vi "array.vi"() -> ()   [LabVIEW 2017]
panel:
  out "Array":T1(array[cluster])
  out "1h avg 2":dbl[][](array[numeric])
  out "24h avg":dbl[][](array[numeric])
  out "Etykiety P1-6":string[][](array[string])
  out "wartosci":i32[](array[numeric])
  out "labels":i32[](array[numeric])
  in  "1h avg":dbl[][](array[numeric])
  out "FuelData":bool
  in  "AvgFuelLabels":T2
  in  "array 2":variant[](array[variant])
  in  "Avg fuel":T3
  in  "dummy fuel array":dbl[][][](array[numeric])
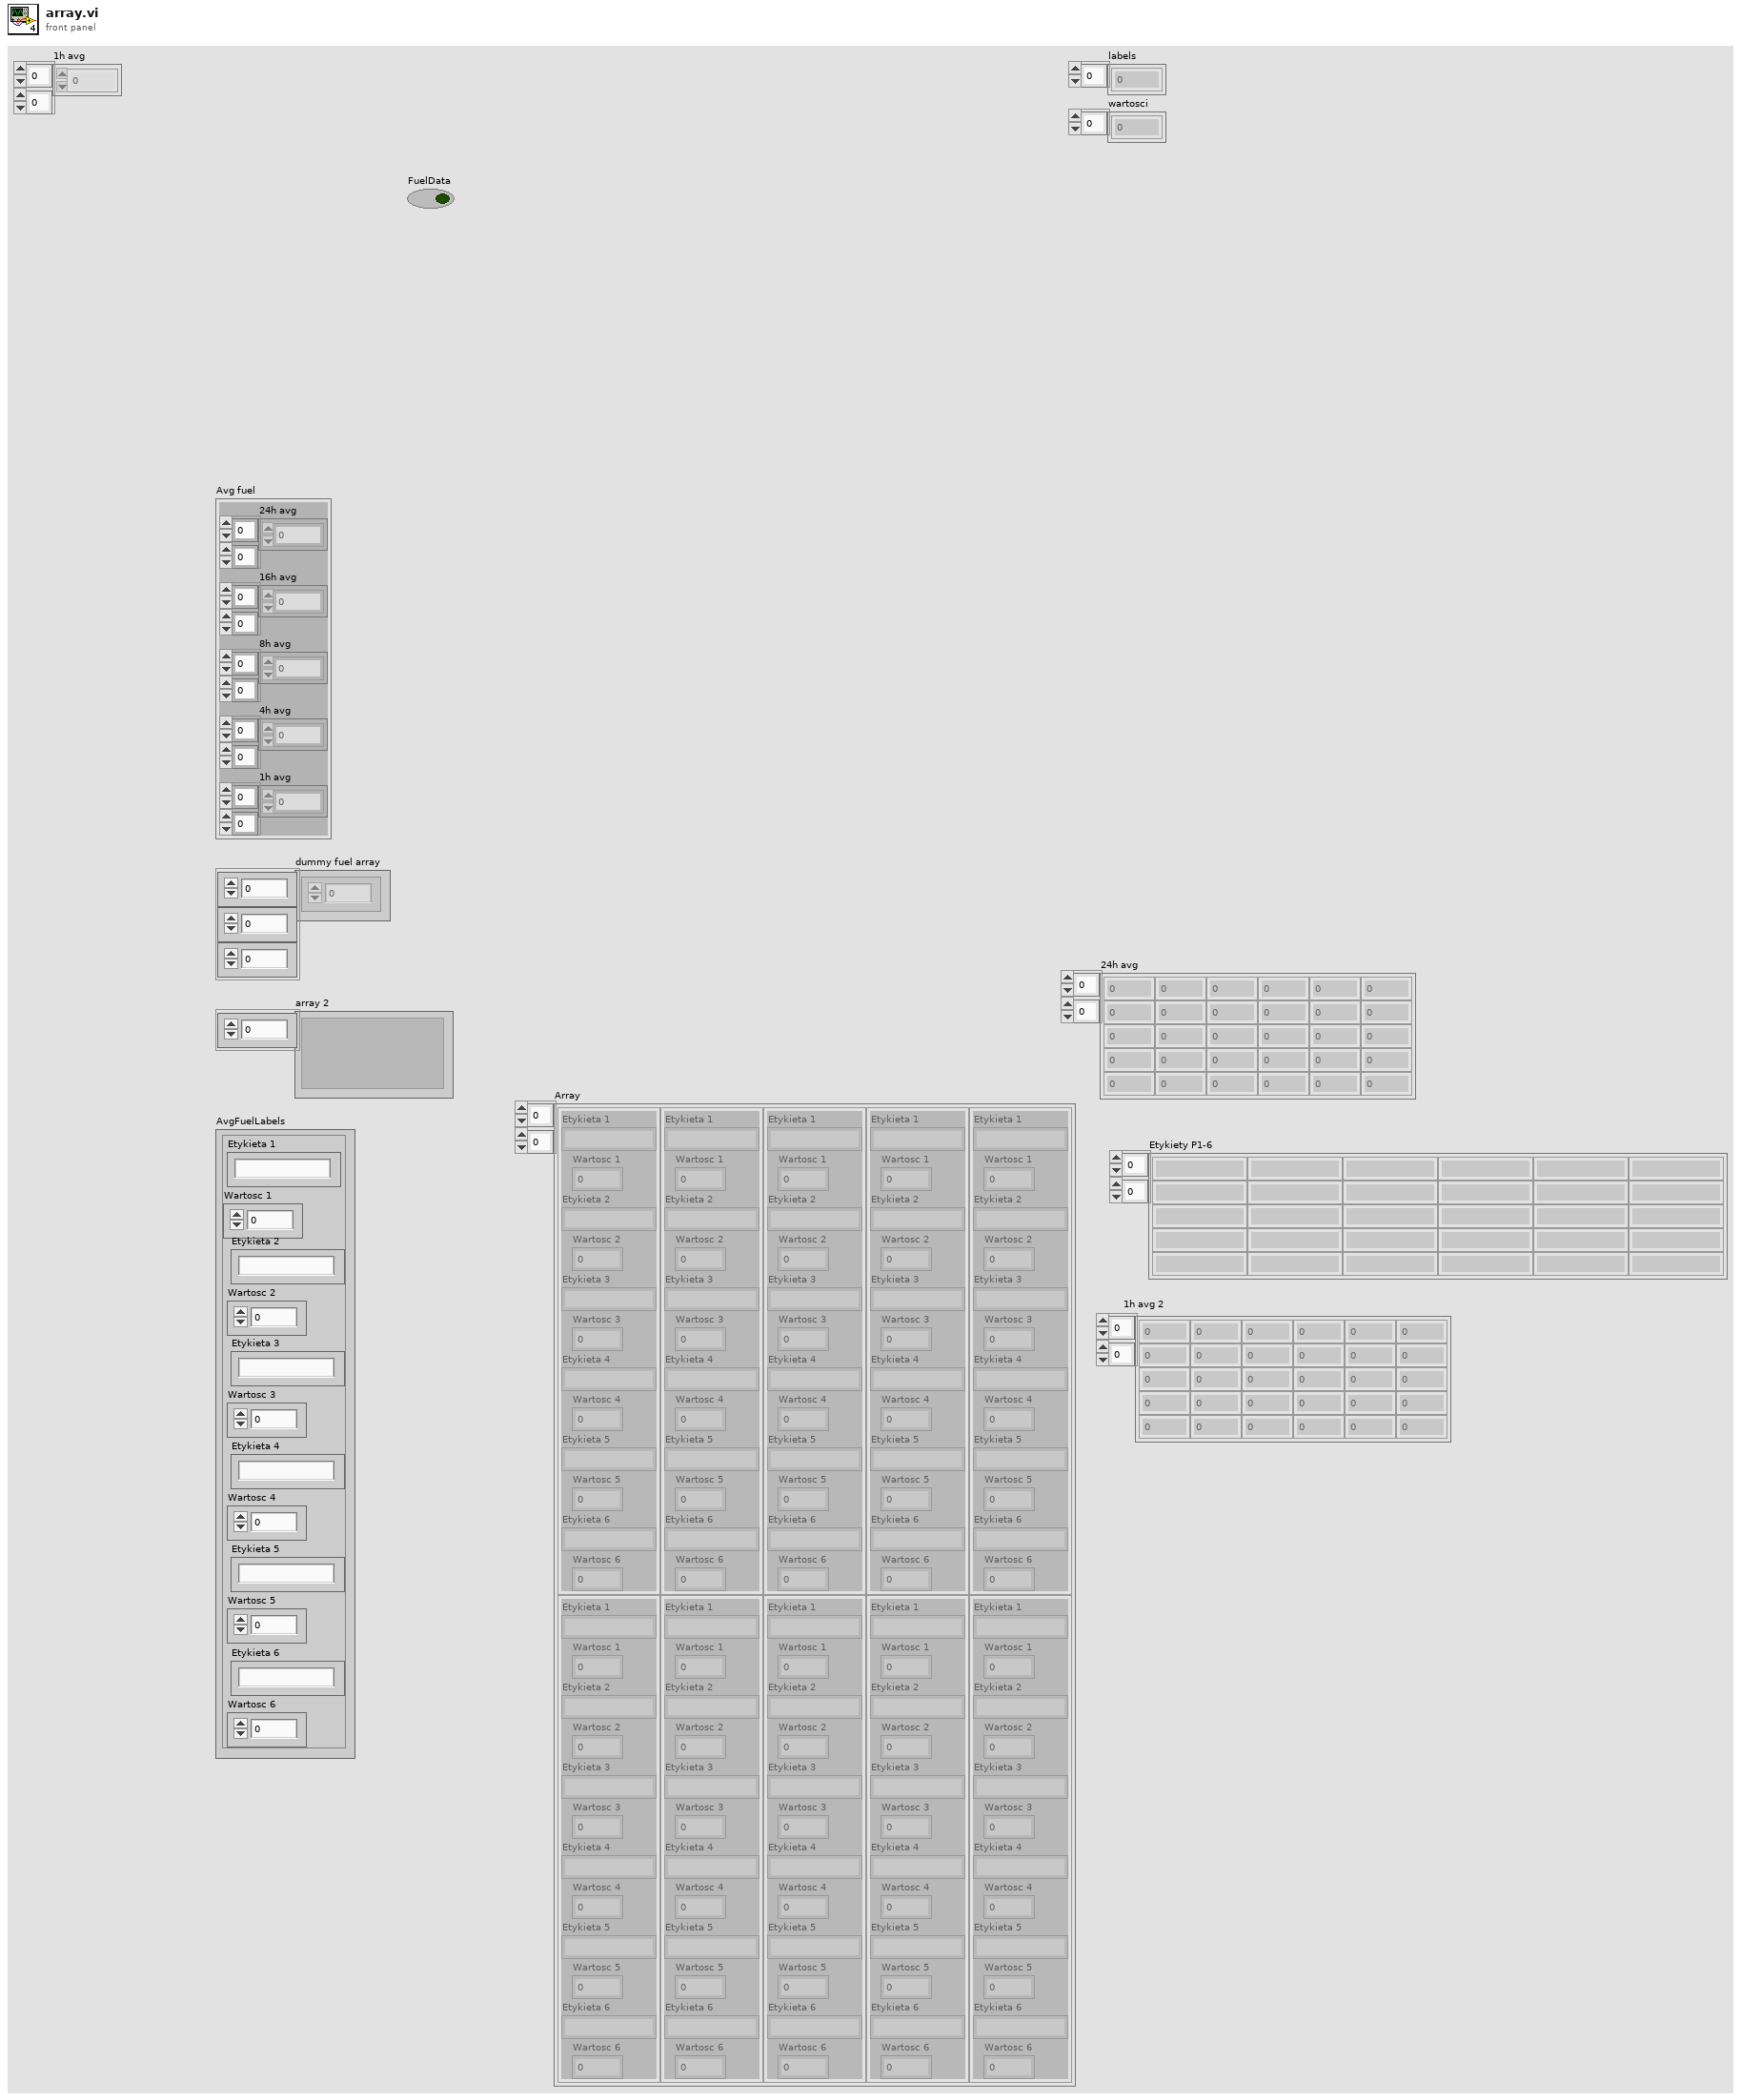
[diagram p1: front panel]
types:
  T1 = cluster{"Etykieta 1":string, "Wartosc 1":dbl, "Etykieta 2":string, "Wartosc 2":dbl, "Etykieta 3":string, "Wartosc 3":dbl, "Etykieta 4":string, "Wartosc 4":dbl, "Etykieta 5":string, "Wartosc 5":dbl, "Etykieta 6":string, "Wartosc 6":dbl}[][]
  T2 = cluster{"Etykieta 1":string, "Wartosc 1":dbl, "Etykieta 2":string, "Wartosc 2":dbl, "Etykieta 3":string, "Wartosc 3":dbl, "Etykieta 4":string, "Wartosc 4":dbl, "Etykieta 5":string, "Wartosc 5":dbl, "Etykieta 6":string, "Wartosc 6":dbl}
  T3 = cluster{"24h avg":dbl[][], "16h avg":dbl[][], "8h avg":dbl[][], "4h avg":dbl[][], "1h avg":dbl[][]}
  T4 = cluster{"Paliwo 1":string, "Paliwo 2":string, "Paliwo 3":string, "Paliwo 4":string, "Paliwo 5":string, "Paliwo 6":string}
  T5 = cluster{"array 2[0]":variant, "array 2[1]":variant, "array 2[2]":variant, "array 2[3]":variant, "array 2[4]":variant, "array 2[5]":variant, "array 2[6]":variant, "array 2[7]":variant, "array 2[8]":variant, "array 2[9]":variant, "array 2[10]":variant, "array 2[11]":variant}
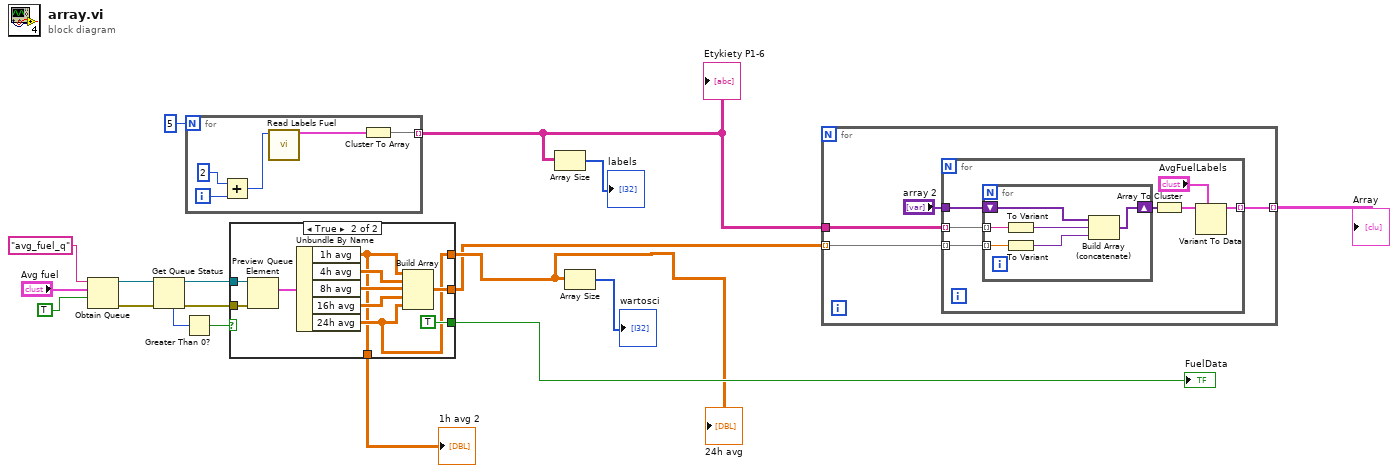
[diagram p0: block diagram]
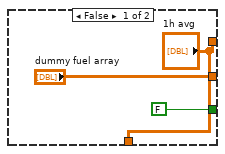
[diagram p2: hidden frame]
diagram:
  n1 = Obtain Queue(name (unnamed)="avg_fuel_q", element data type="Avg fuel", create if not found? (T)=TRUE) -> (queue out=w14:refnum<queue>, error out=w15:errorcluster)  [unwired: 2 in, 1 out]
  n2 = Get Queue Status(queue=w14, error in (no error)=w15) -> (queue out=w12:refnum<queue>, error out=w11:errorcluster, # elements in queue=w9:i32)  [unwired: 1 in, 5 out]
  n3 = Greater Than 0?(x=w9) -> (x > 0?=w10:bool)
  n4 = for {
    N: 5 -> [_]
    tunnel: [w20] -> w4 mode=indexing
    i -> [w23]
    n5 = Add(x=2, y=w23) -> (x+y=w21:i32)
    n6 = call "Read Labels Fuel.vi"("Slave ID"=w21) -> ("Etykiety P1-6"=w19:T4)  [unwired: 10 in]
    n7 = Cluster To Array(cluster=w19) -> (array=w20:string[])
  }
  "Etykiety P1-6" <- w4
  n8 = case shown="True" w10 {
    tunnel: w12 -> [_ w36]
    tunnel: w11 -> [_ w35]
    tunnel: [FALSE TRUE] -> w16
    tunnel: ["dummy fuel array" w33] -> w2
    tunnel: ["1h avg" w28] -> w3
    tunnel: ["1h avg" w27] -> w1
    frame False {
    }
    frame True {
      n9 = Preview Queue Element(queue=w36, error in (no error)=w35) -> (element=w32:T3)  [unwired: 1 in, 3 out]
      n10 = Unbundle By Name(w32) -> ("1h avg"=w27:dbl[][], "4h avg"=w30:dbl[][], "8h avg"=w31:dbl[][], "16h avg"=w29:dbl[][], "24h avg"=w28:dbl[][])
      n11 = Build Array(w27, w30, w31, w29, w28) -> (w33:dbl[][][])
    }
  }
  "FuelData" <- w16
  "24h avg" <- w3
  "1h avg 2" <- w1
  n12 = Array Size(array=w4) -> (size(s)=→"labels":i32[])
  n13 = Array Size(array=w3) -> (size(s)=→"wartosci":i32[])
  n14 = for {
    tunnel: [w40] -> w7 mode=indexing
    tunnel: w4 -> [w38]
    tunnel: w2 -> [w37] mode=indexing
    n15 = for {
      tunnel: w37 -> [w46] mode=indexing
      tunnel: w38 -> [w47] mode=indexing
      tunnel: "array 2" -> [w45]
      tunnel: [w41] -> w40 mode=indexing
      n16 = for {
        tunnel: w47 -> [w52] mode=indexing
        tunnel: w46 -> [w53] mode=indexing
        shift-right: [w50] -> w44
        shift-left: w45 -> [w51]
        n17 = To Variant(anything=w52) -> (Variant=w49:variant)
        n18 = To Variant(anything=w53) -> (Variant=w48:variant)
        n19 = Build Array (concatenate)(w51, w49, w48) -> (w50:variant[])
      }
      n20 = Array To Cluster(array=w44) -> (cluster=w43:T5)
      n21 = Variant To Data(type="AvgFuelLabels", Variant=w43) -> (data=w41:T2)  [unwired: 1 in, 1 out]
    }
  }
  "Array" <- w7
